vi "SP_Breakdown Summery Monthwise_.vi"() -> ()   [LabVIEW 2017]
uses:
  <vilib>/Math Plots/3D Math Plots/3D Pie/3D Pie XCtrl/3D Pie.xctl
  <vilib>/addons/database/Connection.llb/DB Tools Open Connec (Path).vi
  <vilib>/Math Plots/3D Math Plots/3D Pie/3D Pie Datatype/Public/Plot Helper (Vector).vi
  <vilib>/addons/database/NI_Database_API.lvlib
  <vilib>/Math Plots/3D Math Plots/3D Pie/3D Pie Datatype/3D Pie Datatype.lvclass
panel:
  in  "Cancel Button - Archive":bool
  in  "Get Rport 2":bool
  in  "Download 2":bool
  out "error out":errorcluster
  out "BD Count":string[][](array[string])
  out "Duration count":string[][](array[string])
  out "O/P 4":string[](array[string])
  out "month":string
  out "Table":string[][](array[string])
  out "Count":string[](array[string])
  out "Station ID":string[](array[string])
  out "Count out":string[](array[string])
  out "Elements Found out":string[](array[string])
  in  "Select Station":string(combo)
  in  "Shift":string(combo)
  out "T":string
  out "P":string
  out "Q":string
  out "M":string
  out "L":string
  out "GL":string
  in  "Select Year":string(combo)
  in  "Select Month":string(combo)
  in  "Tab Control":T1(tab)
  out "Table Control":string[][](table)
  out "heading 6":string="Total"
  out "heading 5":string="Production"
  out "heading 4":string="Qaulity"
  out "heading 3":string="Maintenance"
  out "heading2":string="Logistics"
  out "heading 1":string="Gap Leader"
  out "Count 2":refnum<class "3D Plot Datatype.lvclass">[](xcontrol)
  out "Duration":refnum<class "3D Plot Datatype.lvclass">[](xcontrol)
  # "Breakdown Summary Report (Month Wise)"
  # "L"
  # "M"
  # "S"
  # "M"
  # "Q"
  # "SS"
  # "TT"
  # "Designed And Developed By - Infinity Automation Systems Pvt. Ltd."
  # "Material"
  # "Safety"
  # "Maintenance"
  # "Quality"
  # "Total"
  # "Date"
  # "Startup/Setup"
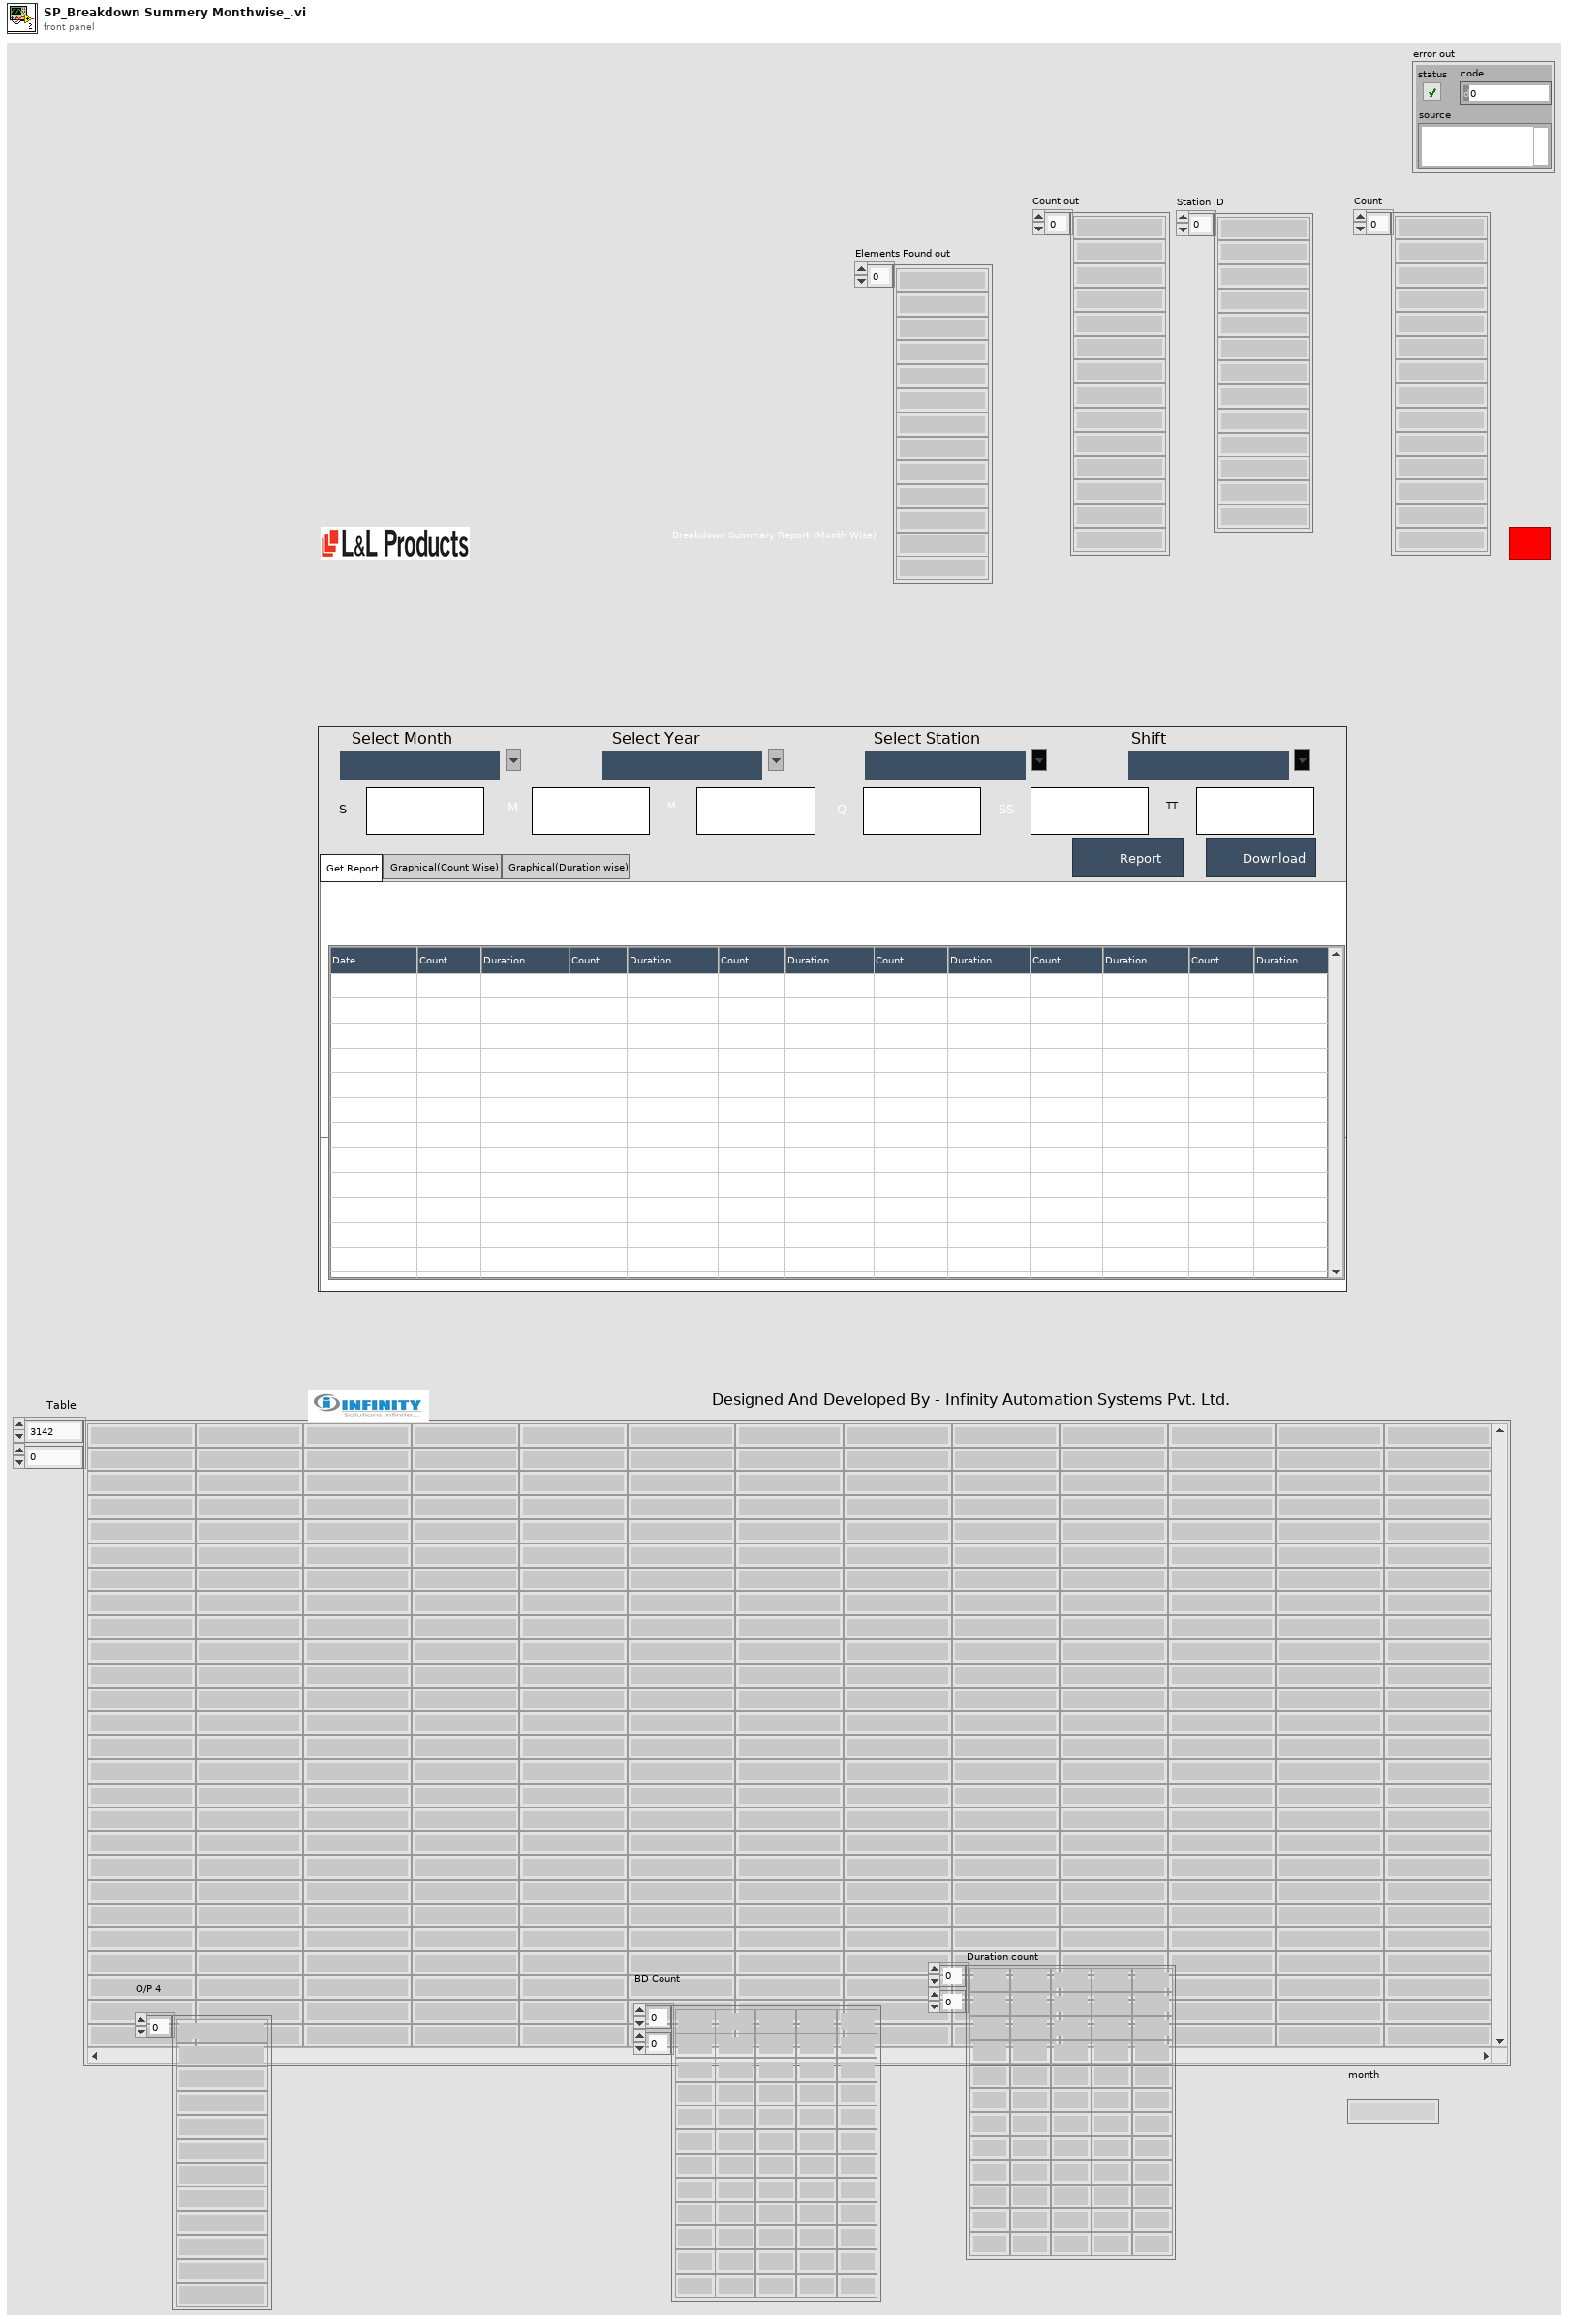
[diagram p1: front panel]
types:
  T1 = enum32{"Get Report", "Graphical(Count Wise) ", "Graphical(Duration wise)"}
  T2 = typedef "NI_Database_API.lvlib/Conn ObjectReference.ctl" = refnum<k1>
  T3 = enum32{"invalid app kind", "Development System", "Run Time System", "Student Edition", "Embedded LabVIEW", "Evaluation", "Custom"}
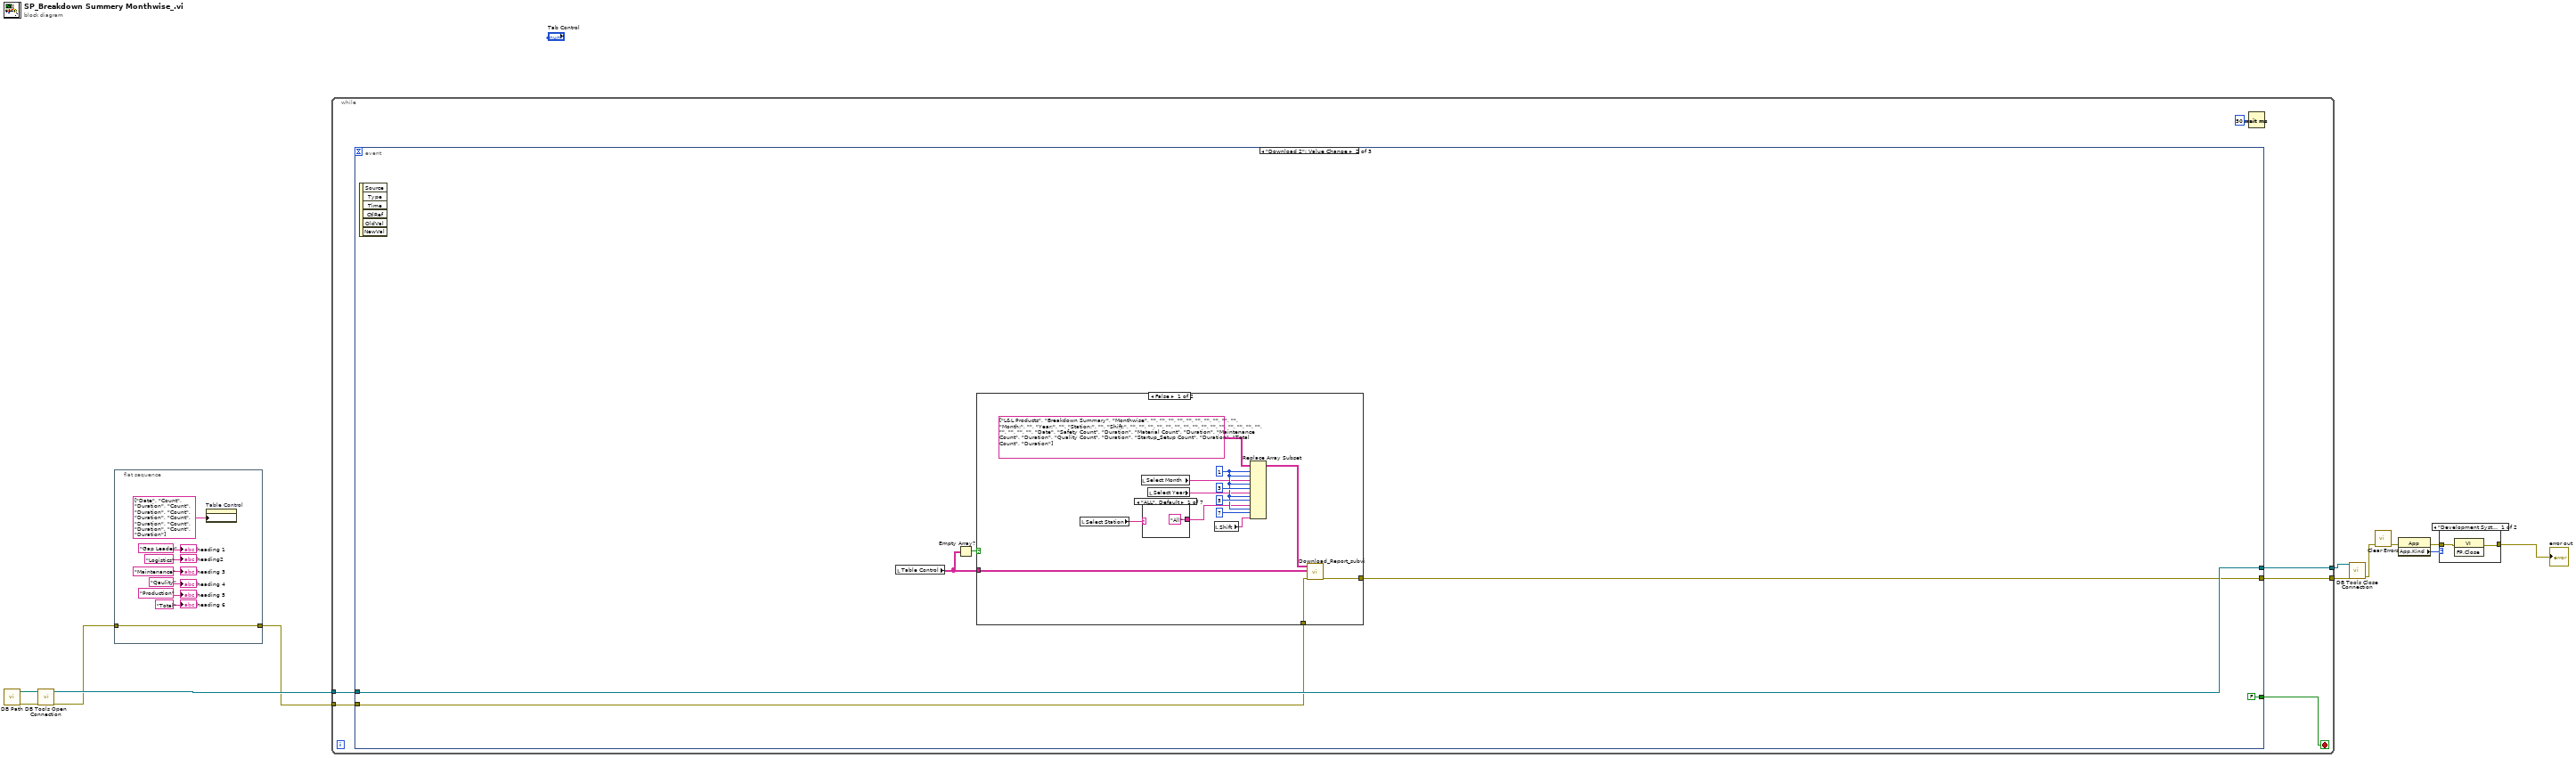
[diagram p0: block diagram]
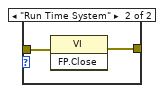
[diagram p2: hidden frame]
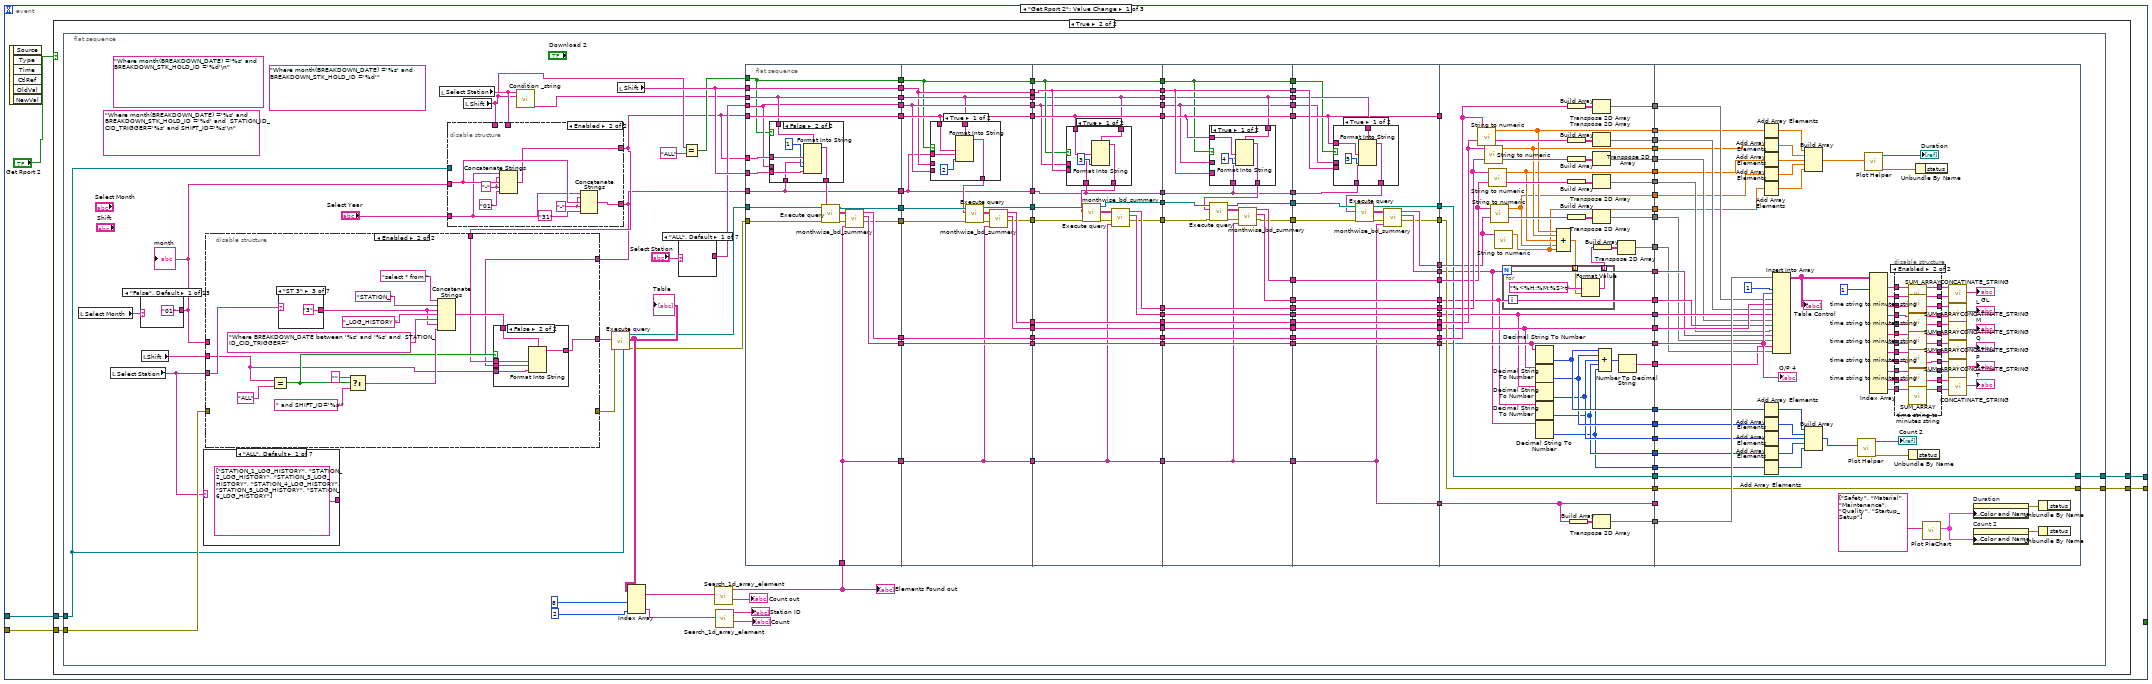
[diagram p3: hidden frame]
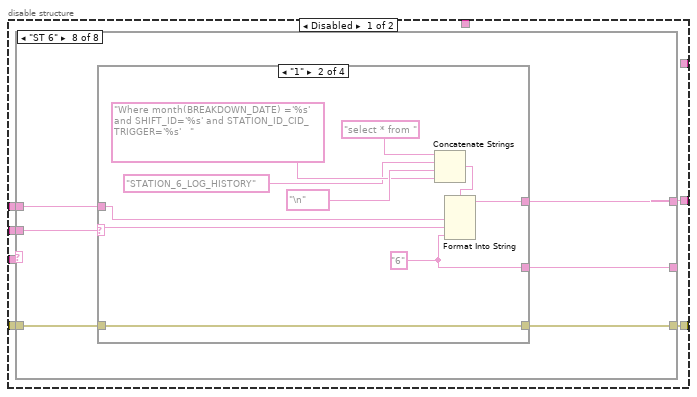
[diagram p5: hidden frame]
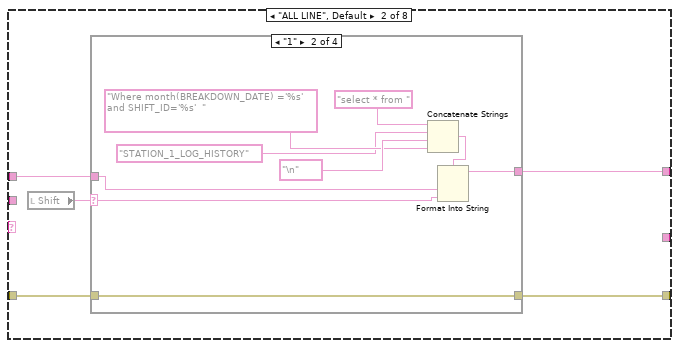
[diagram p7: hidden frame]
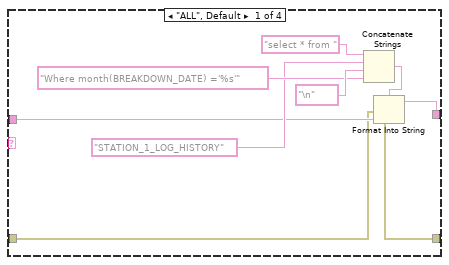
[diagram p8: hidden frame]
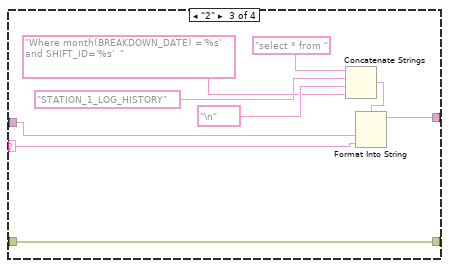
[diagram p9: hidden frame]
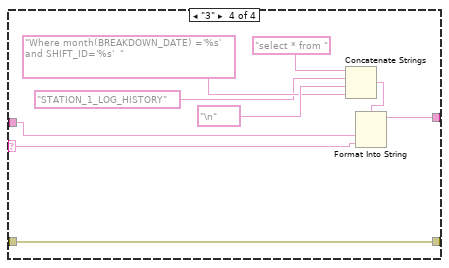
[diagram p10: hidden frame]
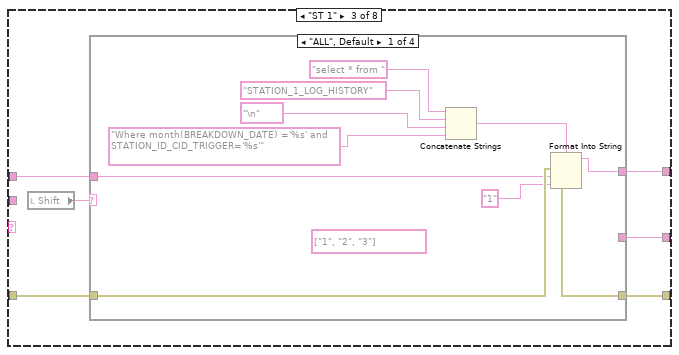
[diagram p11: hidden frame]
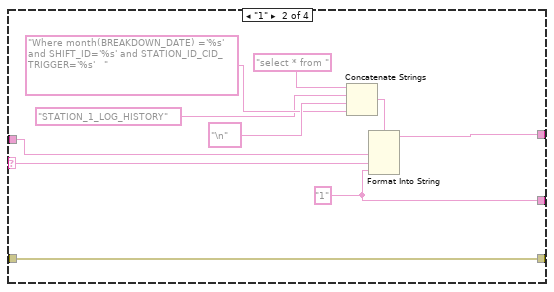
[diagram p12: hidden frame]
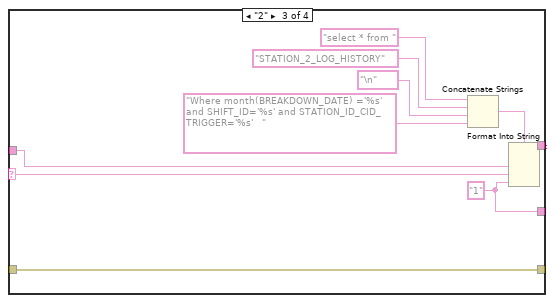
[diagram p13: hidden frame]
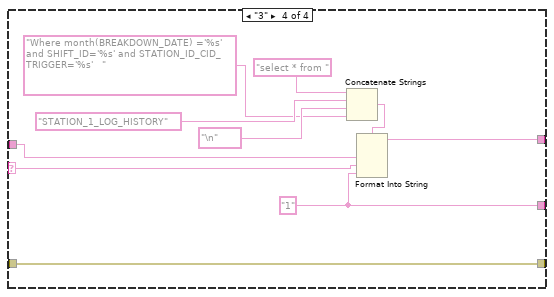
[diagram p14: hidden frame]
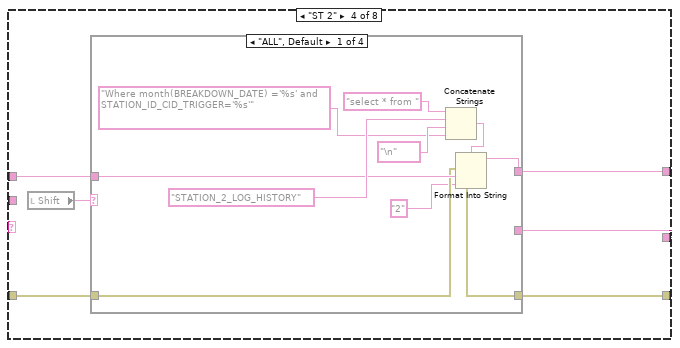
[diagram p15: hidden frame]
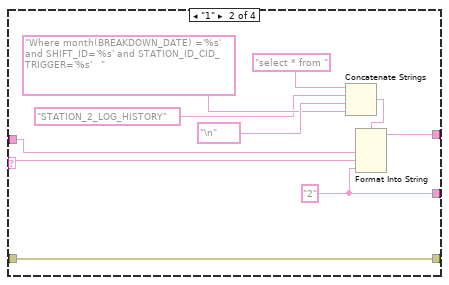
[diagram p16: hidden frame]
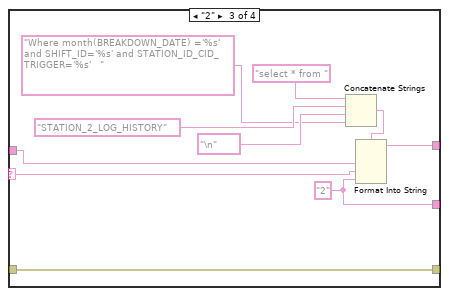
[diagram p17: hidden frame]
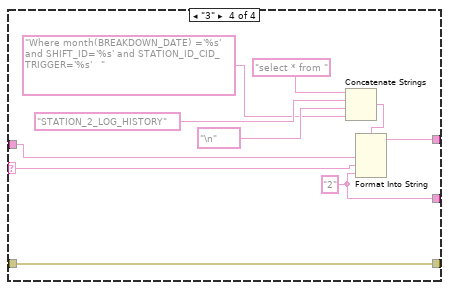
[diagram p18: hidden frame]
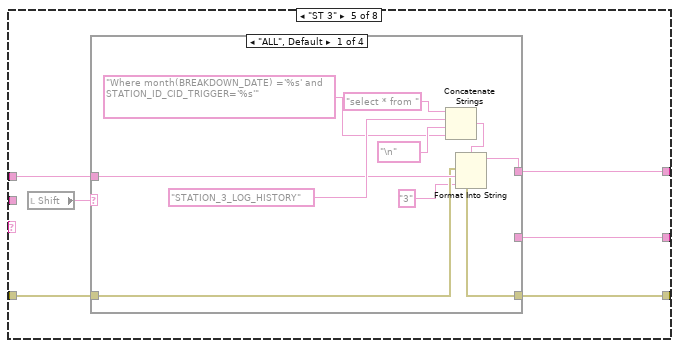
[diagram p19: hidden frame]
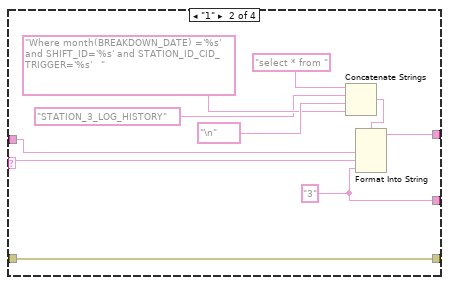
[diagram p20: hidden frame]
diagram:
  n1 = call "DB Path.vi"() -> ("error out"=w12:errorcluster, "DB Path"=w11:path)  [unwired: 10 in]
  n2 = call-poly <vilib>:"DB Tools Open Connection.vi"("error in (no error)"=w12, "connection information"=w11) -> ("error out"=w2:errorcluster, "connection reference"=w10:T2)  [unwired: 6 in]
  n3 = flat-sequence {
    tunnel: [w13] -> w1
    tunnel: w2 -> [w13]
    frame #0 {
      n4 = property on="Table Control" class="Tbl (strict)"("Column Headers[]"=string[] ["Date", "Count", "Duration", "Count", "Duration", "Count", "Duration", "Count", "Duration", "Count", "Duration", "Count", "Duration"] ("Column Header Strings[]")) -> ()  [unwired: 2 in, 2 out]
      "heading 1" <- "Gap Leader" ("heading 1")
      "heading2" <- "Logistics" ("heading2")
      "heading 3" <- "Maintenance" ("heading 3")
      "heading 4" <- "Qaulity" ("heading 4")
      "heading 5" <- "Production" ("heading 5")
      "heading 6" <- "Total" ("heading 6")
    }
  }
  n5 = while {
    tunnel: w1 -> [w26]
    tunnel: w10 -> [w25]
    tunnel: [w23] -> w4
    tunnel: [w22] -> w5
    stop <- w24 stop-if-true
    n6 = event shown="[1] \"Download 2\": Value Change" {
      selector: _ -> [_ _ _]
      dyn-events: _ -> [_ _ _]
      timeout: _ -> [_ _ _]
      tunnel: w26 -> [w31 w890 w917]
      tunnel: w25 -> [w30 w892 w916]
      tunnel: [_ FALSE ("Cancel Button - Archive") "Cancel Button - Archive"] -> w24
      tunnel: [w29 w889 w917] -> w23
      tunnel: [w28 w892 w916] -> w22
      event "Get Rport 2": Value Change {
        n7 = event-data() -> ()  [unwired: 1 in, 6 out]
        n8 = case shown="True" "Get Rport 2" {
          tunnel: w31 -> [_ w35]
          tunnel: w30 -> [_ w34]
          tunnel: [_ w33] -> w29
          tunnel: [_ w32] -> w28
          frame False {
          }
          frame True {
            n9 = flat-sequence {
              tunnel: w35 -> [w159]
              tunnel: w34 -> [w66]
              tunnel: [w63] -> w33
              tunnel: [w61] -> w32
              frame #0 {
                (unwired) "Where month(BREAKDOWN_DATE) ='%s' and  BREAKDOWN_STK_HOLD_ID ='%d' and  STATION_ID_CID_TRIGGER='%s' and SHIFT_ID='%s'\n" ("condition")
                (unwired) "Where month(BREAKDOWN_DATE) ='%s' and  BREAKDOWN_STK_HOLD_ID ='%d'" ("condition")
                (unwired) "Where month(BREAKDOWN_DATE) ='%s' and  BREAKDOWN_STK_HOLD_ID ='%d'\n" ("condition")
                n10 = local read "Select Month"() -> (w156:string)
                n11 = local read "Select Station"() -> (w57:string)
                n12 = case shown="\"False\", Default" w156 {
                  tunnel: ["01" "01" "02" "03" "04" "05" "06" "07" "08" "09" "10" "11" "12"] -> w65
                  frame "False", Default {
                  }
                  frame "January" {
                  }
                  frame "February" {
                  }
                  frame "March" {
                  }
                  frame "April" {
                  }
                  frame "May" {
                  }
                  frame "June" {
                  }
                  frame "July" {
                  }
                  frame "August" {
                  }
                  frame "September" {
                  }
                  frame "October" {
                  }
                  frame "November" {
                  }
                  frame "December" {
                  }
                }
                "month" <- w65
                n13 = local read "Shift"() -> (w48:string)
                n14 = case shown="\"ALL\", Default" w57 {
                  tunnel: [string[] ["STATION_1_LOG_HISTORY", "STATION_2_LOG_HISTORY", "STATION_3_LOG_HISTORY", "STATION_4_LOG_HISTORY", "STATION_5_LOG_HISTORY", "STATION_6_LOG_HISTORY"] string[] ["STATION_1_LOG_HISTORY"] string[] ["STATION_2_LOG_HISTORY"] string[] ["STATION_3_LOG_HISTORY"] string[] ["STATION_4_LOG_HISTORY"] string[] ["STATION_5_LOG_HISTORY"] string[] ["STATION_6_LOG_HISTORY"]] -> _
                  frame "ALL", Default {
                  }
                  frame "STATION 1" {
                  }
                  frame "STATION 2" {
                  }
                  frame "STATION 3" {
                  }
                  frame "STATION 4" {
                  }
                  frame "STATION 5" {
                  }
                  frame "STATION 6" {
                  }
                }
                n15 = local read "Select Station"() -> (w67:string)
                n16 = local read "Shift"() -> (w56:string)
                n17 = disable-structure shown="Enabled" {
                  disable-tunnel: w67 -> [w538 _]
                  disable-tunnel: w66 -> [w537 _]
                  disable-tunnel: w56 -> [w536 _]
                  disable-tunnel: w65 -> [w535 w546]
                  disable-tunnel: "Select Year" -> [w534 w539]
                  disable-tunnel: [_ w545] -> w47
                  disable-tunnel: [_ w544] -> w46
                  frame Disabled {
                    # "T=2\nF=4"
                    n18 = call "Condition _string_For_Month.vi"("Select Line 2"=w538, "connection reference"=w537, "Shift"=w536, "year"=w534, "month"=w535) -> ("Duration count"=→"Duration count":string[][], "BD Count"=→"BD Count":string[][])  [unwired: 11 in, 2 out]
                  }
                  frame Enabled {
                    w540 = "-" ("string")
                    w541 = "-" ("string")
                    n19 = Concatenate Strings(w539, w541, w546, w541, "01" ("string")) -> (w545:string)
                    n20 = Concatenate Strings(w539, w540, w546, w540, "31" ("string")) -> (w544:string)
                  }
                }
                n21 = disable-structure shown="Enabled" {
                  disable-tunnel: [w169 w487] -> w163
                  disable-tunnel: w159 -> [w168 _]
                  disable-tunnel: [w167 _] -> w158
                  disable-tunnel: w65 -> [w166 _]
                  disable-tunnel: w57 -> [w165 w494]
                  disable-tunnel: w48 -> [w164 w488]
                  disable-tunnel: w47 -> [_ w490]
                  disable-tunnel: w46 -> [_ w489]
                  frame Disabled {
                    n22 = case shown="\"ST 6\"" w165 {
                      tunnel: w166 -> [_ w174 w216 w262 w308 w354 w400 w446]
                      tunnel: [_ w173 w215 w261 w307 w353 w399 w445] -> w169
                      tunnel: w168 -> [_ w172 w214 w260 w306 w352 w398 w444]
                      tunnel: [_ w171 w213 w259 w305 w351 w397 w443] -> w167
                      tunnel: [_ _ w211 w257 w303 w349 w395 w442] -> _
                      tunnel: w164 -> [_ _ _ _ _ _ _ w441]
                      frame "False" {
                      }
                      frame "ALL LINE", Default {
                        n23 = local read "Shift"() -> (w170:string)
                        n24 = case shown="\"1\"" w170 {
                          selector: w170 -> [_ w185 w194 w203]
                          tunnel: [w179 w188 w197 w206] -> w173
                          tunnel: [w178 w184 w193 w202] -> w171
                          tunnel: w174 -> [w176 w186 w195 w204]
                          tunnel: w172 -> [w175 w184 w193 w202]
                          frame "ALL", Default {
                            n25 = Concatenate Strings("select * from " ("string"), "STATION_1_LOG_HISTORY" ("table"), "\n" ("string"), "Where month(BREAKDOWN_DATE) ='%s'" ("condition")) -> (w180:string)
                            n26 = Format Into String(format string=w180, error in=w175, w176) -> (resulting string=w179:string, error out=w178:errorcluster)  [unwired: 1 in]
                          }
                          frame "1" {
                            n27 = Concatenate Strings("select * from " ("string"), "STATION_1_LOG_HISTORY" ("table"), "\n" ("string"), "Where month(BREAKDOWN_DATE) ='%s' and SHIFT_ID='%s'  " ("condition")) -> (w190:string)
                            n28 = Format Into String(format string=w190, w186, w185) -> (resulting string=w188:string)  [unwired: 2 in, 1 out]
                          }
                          frame "2" {
                            n29 = Concatenate Strings("select * from " ("string"), "STATION_1_LOG_HISTORY" ("table"), "\n" ("string"), "Where month(BREAKDOWN_DATE) ='%s' and SHIFT_ID='%s'  " ("condition")) -> (w199:string)
                            n30 = Format Into String(format string=w199, w195, w194) -> (resulting string=w197:string)  [unwired: 2 in, 1 out]
                          }
                          frame "3" {
                            n31 = Concatenate Strings("select * from " ("string"), "STATION_1_LOG_HISTORY" ("table"), "\n" ("string"), "Where month(BREAKDOWN_DATE) ='%s' and SHIFT_ID='%s'  " ("condition")) -> (w208:string)
                            n32 = Format Into String(format string=w208, w204, w203) -> (resulting string=w206:string)  [unwired: 2 in, 1 out]
                          }
                        }
                      }
                      frame "ST 1" {
                        n33 = local read "Shift"() -> (w212:string)
                        n34 = case shown="\"ALL\", Default" w212 {
                          selector: w212 -> [_ w230 w240 w250]
                          tunnel: [w222 w233 w243 w253] -> w215
                          tunnel: [w221 w229 w239 w249] -> w213
                          tunnel: w216 -> [w217 w231 w241 w251]
                          tunnel: w214 -> [w219 w229 w239 w249]
                          tunnel: [_ w227 w237 w247] -> w211
                          frame "ALL", Default {
                            (unwired) string[] ["1", "2", "3"]
                            n35 = Concatenate Strings("select * from " ("string"), "STATION_1_LOG_HISTORY" ("table"), "\n" ("string"), "Where month(BREAKDOWN_DATE) ='%s' and  STATION_ID_CID_TRIGGER='%s'" ("condition")) -> (w223:string)
                            n36 = Format Into String(format string=w223, error in=w219, w217, "1") -> (resulting string=w222:string, error out=w221:errorcluster)  [unwired: 1 in]
                          }
                          frame "1" {
                            w227 = "1"
                            n37 = Concatenate Strings("select * from " ("string"), "STATION_1_LOG_HISTORY" ("table"), "\n" ("string"), "Where month(BREAKDOWN_DATE) ='%s' and SHIFT_ID='%s' and STATION_ID_CID_TRIGGER='%s'   " ("condition")) -> (w228:string)
                            n38 = Format Into String(format string=w228, w231, w230, w227) -> (resulting string=w233:string)  [unwired: 2 in, 1 out]
                          }
                          frame "2" {
                            w237 = "1" ("input 3")
                            n39 = Concatenate Strings("select * from " ("string"), "STATION_2_LOG_HISTORY" ("table"), "\n" ("string"), "Where month(BREAKDOWN_DATE) ='%s' and SHIFT_ID='%s' and STATION_ID_CID_TRIGGER='%s'   " ("condition")) -> (w244:string)
                            n40 = Format Into String(format string=w244, w241, w240, w237) -> (resulting string=w243:string)  [unwired: 2 in, 1 out]
                          }
                          frame "3" {
                            w247 = "1" ("input 3")
                            n41 = Concatenate Strings("select * from " ("string"), "STATION_1_LOG_HISTORY" ("table"), "\n" ("string"), "Where month(BREAKDOWN_DATE) ='%s' and SHIFT_ID='%s' and STATION_ID_CID_TRIGGER='%s'   " ("condition")) -> (w254:string)
                            n42 = Format Into String(format string=w254, w251, w250, w247) -> (resulting string=w253:string)  [unwired: 2 in, 1 out]
                          }
                        }
                      }
                      frame "ST 2" {
                        n43 = local read "Shift"() -> (w258:string)
                        n44 = case shown="\"ALL\", Default" w258 {
                          selector: w258 -> [_ w275 w286 w296]
                          tunnel: [w269 w278 w289 w299] -> w261
                          tunnel: [w268 w274 w285 w295] -> w259
                          tunnel: w262 -> [w266 w276 w287 w297]
                          tunnel: w260 -> [w265 w274 w285 w295]
                          tunnel: [_ w273 w283 w293] -> w257
                          frame "ALL", Default {
                            n45 = Concatenate Strings("select * from " ("string"), "STATION_2_LOG_HISTORY" ("table"), "\n" ("string"), "Where month(BREAKDOWN_DATE) ='%s' and  STATION_ID_CID_TRIGGER='%s'" ("condition")) -> (w270:string)
                            n46 = Format Into String(format string=w270, error in=w265, w266, "2" ("input 2")) -> (resulting string=w269:string, error out=w268:errorcluster)  [unwired: 1 in]
                          }
                          frame "1" {
                            w273 = "2"
                            n47 = Concatenate Strings("select * from " ("string"), "STATION_2_LOG_HISTORY" ("table"), "\n" ("string"), "Where month(BREAKDOWN_DATE) ='%s' and SHIFT_ID='%s' and STATION_ID_CID_TRIGGER='%s'   " ("condition")) -> (w280:string)
                            n48 = Format Into String(format string=w280, w276, w275, w273) -> (resulting string=w278:string)  [unwired: 2 in, 1 out]
                          }
                          frame "2" {
                            w283 = "2" ("input 3")
                            n49 = Concatenate Strings("select * from " ("string"), "STATION_2_LOG_HISTORY" ("table"), "\n" ("string"), "Where month(BREAKDOWN_DATE) ='%s' and SHIFT_ID='%s' and STATION_ID_CID_TRIGGER='%s'   " ("condition")) -> (w290:string)
                            n50 = Format Into String(format string=w290, w287, w286, w283) -> (resulting string=w289:string)  [unwired: 2 in, 1 out]
                          }
                          frame "3" {
                            w293 = "2" ("input 3")
                            n51 = Concatenate Strings("select * from " ("string"), "STATION_2_LOG_HISTORY" ("table"), "\n" ("string"), "Where month(BREAKDOWN_DATE) ='%s' and SHIFT_ID='%s' and STATION_ID_CID_TRIGGER='%s'   " ("condition")) -> (w300:string)
                            n52 = Format Into String(format string=w300, w297, w296, w293) -> (resulting string=w299:string)  [unwired: 2 in, 1 out]
                          }
                        }
                      }
                      frame "ST 3" {
                        n53 = local read "Shift"() -> (w304:string)
                        n54 = case shown="\"ALL\", Default" w304 {
                          selector: w304 -> [_ w321 w332 w342]
                          tunnel: [w315 w324 w335 w345] -> w307
                          tunnel: [w314 w320 w331 w341] -> w305
                          tunnel: w308 -> [w312 w322 w333 w343]
                          tunnel: w306 -> [w311 w320 w331 w341]
                          tunnel: [_ w319 w329 w339] -> w303
                          frame "ALL", Default {
                            n55 = Concatenate Strings("select * from " ("string"), "STATION_3_LOG_HISTORY" ("table"), "\n" ("string"), "Where month(BREAKDOWN_DATE) ='%s' and  STATION_ID_CID_TRIGGER='%s'" ("condition")) -> (w316:string)
                            n56 = Format Into String(format string=w316, error in=w311, w312, "3" ("input 2")) -> (resulting string=w315:string, error out=w314:errorcluster)  [unwired: 1 in]
                          }
                          frame "1" {
                            w319 = "3"
                            n57 = Concatenate Strings("select * from " ("string"), "STATION_3_LOG_HISTORY" ("table"), "\n" ("string"), "Where month(BREAKDOWN_DATE) ='%s' and SHIFT_ID='%s' and STATION_ID_CID_TRIGGER='%s'   " ("condition")) -> (w326:string)
                            n58 = Format Into String(format string=w326, w322, w321, w319) -> (resulting string=w324:string)  [unwired: 2 in, 1 out]
                          }
                          frame "2" {
                            w329 = "3" ("input 3")
                            n59 = Concatenate Strings("select * from " ("string"), "STATION_3_LOG_HISTORY" ("table"), "\n" ("string"), "Where month(BREAKDOWN_DATE) ='%s' and SHIFT_ID='%s' and STATION_ID_CID_TRIGGER='%s'   " ("condition")) -> (w336:string)
                            n60 = Format Into String(format string=w336, w333, w332, w329) -> (resulting string=w335:string)  [unwired: 2 in, 1 out]
                          }
                          frame "3" {
                            w339 = "3" ("input 3")
                            n61 = Concatenate Strings("select * from " ("string"), "STATION_3_LOG_HISTORY" ("table"), "\n" ("string"), "Where month(BREAKDOWN_DATE) ='%s' and SHIFT_ID='%s' and STATION_ID_CID_TRIGGER='%s'   " ("condition")) -> (w346:string)
                            n62 = Format Into String(format string=w346, w343, w342, w339) -> (resulting string=w345:string)  [unwired: 2 in, 1 out]
                          }
                        }
                      }
                      frame "ST 4" {
                        n63 = local read "Shift"() -> (w350:string)
                        n64 = case shown="\"ALL\", Default" w350 {
                          selector: w350 -> [_ w367 w378 w388]
                          tunnel: [w361 w370 w381 w391] -> w353
                          tunnel: [w360 w366 w377 w387] -> w351
                          tunnel: w354 -> [w358 w368 w379 w389]
                          tunnel: w352 -> [w357 w366 w377 w387]
                          tunnel: [_ w365 w375 w385] -> w349
                          frame "ALL", Default {
                            n65 = Concatenate Strings("select * from " ("string"), "STATION_4_LOG_HISTORY" ("table"), "\n" ("string"), "Where month(BREAKDOWN_DATE) ='%s' and  STATION_ID_CID_TRIGGER='%s'" ("condition")) -> (w362:string)
                            n66 = Format Into String(format string=w362, error in=w357, w358, "4" ("input 2")) -> (resulting string=w361:string, error out=w360:errorcluster)  [unwired: 1 in]
                          }
                          frame "1" {
                            w365 = "4"
                            n67 = Concatenate Strings("select * from " ("string"), "STATION_4_LOG_HISTORY" ("table"), "\n" ("string"), "Where month(BREAKDOWN_DATE) ='%s' and SHIFT_ID='%s' and STATION_ID_CID_TRIGGER='%s'   " ("condition")) -> (w372:string)
                            n68 = Format Into String(format string=w372, w368, w367, w365) -> (resulting string=w370:string)  [unwired: 2 in, 1 out]
                          }
                          frame "2" {
                            w375 = "4" ("input 3")
                            n69 = Concatenate Strings("select * from " ("string"), "STATION_4_LOG_HISTORY" ("table"), "\n" ("string"), "Where month(BREAKDOWN_DATE) ='%s' and SHIFT_ID='%s' and STATION_ID_CID_TRIGGER='%s'   " ("condition")) -> (w382:string)
                            n70 = Format Into String(format string=w382, w379, w378, w375) -> (resulting string=w381:string)  [unwired: 2 in, 1 out]
                          }
                          frame "3" {
                            w385 = "4" ("input 3")
                            n71 = Concatenate Strings("select * from " ("string"), "STATION_4_LOG_HISTORY" ("table"), "\n" ("string"), "Where month(BREAKDOWN_DATE) ='%s' and SHIFT_ID='%s' and STATION_ID_CID_TRIGGER='%s'   " ("condition")) -> (w392:string)
                            n72 = Format Into String(format string=w392, w389, w388, w385) -> (resulting string=w391:string)  [unwired: 2 in, 1 out]
                          }
                        }
                      }
                      frame "ST 5" {
                        n73 = local read "Shift"() -> (w396:string)
                        n74 = case shown="\"ALL\", Default" w396 {
                          selector: w396 -> [_ w413 w424 w434]
                          tunnel: [w407 w416 w427 w437] -> w399
                          tunnel: [w406 w412 w423 w433] -> w397
                          tunnel: w400 -> [w404 w414 w425 w435]
                          tunnel: w398 -> [w403 w412 w423 w433]
                          tunnel: [_ w411 w421 w431] -> w395
                          frame "ALL", Default {
                            n75 = Concatenate Strings("select * from " ("string"), "STATION_5_LOG_HISTORY" ("table"), "\n" ("string"), "Where month(BREAKDOWN_DATE) ='%s' and  STATION_ID_CID_TRIGGER='%s'" ("condition")) -> (w408:string)
                            n76 = Format Into String(format string=w408, error in=w403, w404, "5" ("input 2")) -> (resulting string=w407:string, error out=w406:errorcluster)  [unwired: 1 in]
                          }
                          frame "1" {
                            w411 = "5"
                            n77 = Concatenate Strings("select * from " ("string"), "STATION_5_LOG_HISTORY" ("table"), "\n" ("string"), "Where month(BREAKDOWN_DATE) ='%s' and SHIFT_ID='%s' and STATION_ID_CID_TRIGGER='%s'   " ("condition")) -> (w418:string)
                            n78 = Format Into String(format string=w418, w414, w413, w411) -> (resulting string=w416:string)  [unwired: 2 in, 1 out]
                          }
                          frame "2" {
                            w421 = "5" ("input 3")
                            n79 = Concatenate Strings("select * from " ("string"), "STATION_5_LOG_HISTORY" ("table"), "\n" ("string"), "Where month(BREAKDOWN_DATE) ='%s' and SHIFT_ID='%s' and STATION_ID_CID_TRIGGER='%s'   " ("condition")) -> (w428:string)
                            n80 = Format Into String(format string=w428, w425, w424, w421) -> (resulting string=w427:string)  [unwired: 2 in, 1 out]
                          }
                          frame "3" {
                            w431 = "5" ("input 3")
                            n81 = Concatenate Strings("select * from " ("string"), "STATION_5_LOG_HISTORY" ("table"), "\n" ("string"), "Where month(BREAKDOWN_DATE) ='%s' and SHIFT_ID='%s' and STATION_ID_CID_TRIGGER='%s'   " ("condition")) -> (w438:string)
                            n82 = Format Into String(format string=w438, w435, w434, w431) -> (resulting string=w437:string)  [unwired: 2 in, 1 out]
                          }
                        }
                      }
                      frame "ST 6" {
                        n83 = case shown="\"1\"" w441 {
                          selector: w441 -> [_ w459 w470 w480]
                          tunnel: [w453 w462 w473 w483] -> w445
                          tunnel: [w452 w458 w469 w479] -> w443
                          tunnel: w446 -> [w450 w460 w471 w481]
                          tunnel: w444 -> [w449 w458 w469 w479]
                          tunnel: [_ w457 w467 w477] -> w442
                          frame "ALL", Default {
                            n84 = Concatenate Strings("select * from " ("string"), "STATION_6_LOG_HISTORY" ("table"), "\n" ("string"), "Where month(BREAKDOWN_DATE) ='%s' and  STATION_ID_CID_TRIGGER='%s'" ("condition")) -> (w454:string)
                            n85 = Format Into String(format string=w454, error in=w449, w450, "6" ("input 2")) -> (resulting string=w453:string, error out=w452:errorcluster)  [unwired: 1 in]
                          }
                          frame "1" {
                            w457 = "6"
                            n86 = Concatenate Strings("select * from " ("string"), "STATION_6_LOG_HISTORY" ("table"), "\n" ("string"), "Where month(BREAKDOWN_DATE) ='%s' and SHIFT_ID='%s' and STATION_ID_CID_TRIGGER='%s'   " ("condition")) -> (w464:string)
                            n87 = Format Into String(format string=w464, w460, w459, w457) -> (resulting string=w462:string)  [unwired: 2 in, 1 out]
                          }
                          frame "2" {
                            w467 = "6" ("input 3")
                            n88 = Concatenate Strings("select * from " ("string"), "STATION_6_LOG_HISTORY" ("table"), "\n" ("string"), "Where month(BREAKDOWN_DATE) ='%s' and SHIFT_ID='%s' and STATION_ID_CID_TRIGGER='%s'   " ("condition")) -> (w474:string)
                            n89 = Format Into String(format string=w474, w471, w470, w467) -> (resulting string=w473:string)  [unwired: 2 in, 1 out]
                          }
                          frame "3" {
                            w477 = "6" ("input 3")
                            n90 = Concatenate Strings("select * from " ("string"), "STATION_6_LOG_HISTORY" ("table"), "\n" ("string"), "Where month(BREAKDOWN_DATE) ='%s' and SHIFT_ID='%s' and STATION_ID_CID_TRIGGER='%s'   " ("condition")) -> (w484:string)
                            n91 = Format Into String(format string=w484, w481, w480, w477) -> (resulting string=w483:string)  [unwired: 2 in, 1 out]
                          }
                        }
                      }
                    }
                  }
                  frame Enabled {
                    n92 = Equal?(x=w488, y="ALL" ("condition")) -> (x = y?=w492:bool)
                    n93 = case shown="\"ST 3\"" w494 {
                      tunnel: ["1" "2" "3" "4" "5" "6" "1"] -> w493
                      frame "ST 1" {
                      }
                      frame "ST 2" {
                      }
                      frame "ST 3" {
                      }
                      frame "ST 4" {
                      }
                      frame "ST 5" {
                      }
                      frame "ST 6" {
                      }
                      frame "ALL", Default {
                      }
                    }
                    n94 = Select(t="", s=w492, f=" and SHIFT_ID='%s'" ("condition")) -> (s? t:f=w502:string)
                    n95 = Concatenate Strings("select * from " ("string"), "STATION_" ("table"), w493, "_LOG_HISTORY " ("table"), "Where BREAKDOWN_DATE between '%s' and '%s' and  STATION_ID_CID_TRIGGER=" ("condition"), w493, w502) -> (w491:string)
                    n96 = case shown="False" w492 {
                      tunnel: w490 -> [w506 w511]
                      tunnel: w491 -> [w505 w510]
                      tunnel: [w504 w509] -> w487
                      tunnel: w489 -> [w503 w508]
                      tunnel: w488 -> [_ w507]
                      frame True {
                        n97 = Format Into String(format string=w505, w506, w503) -> (resulting string=w504:string)  [unwired: 2 in, 1 out]
                      }
                      frame False {
                        n98 = Format Into String(format string=w510, w511, w508, w507) -> (resulting string=w509:string)  [unwired: 2 in, 1 out]
                      }
                    }
                  }
                }
                n99 = call "Condition _string.vi"("Shift"=w56, "Select Line 2"=w67) -> ("String"=w53:string)  [unwired: 7 in, 2 out]
                n100 = call "Execute query.vi"("error in (no error)"=w158, "String"=w163, "connection reference"=w66) -> ("error out"=w151:errorcluster, "Table"=w161:string[][], "connection reference 2"=w150:T2)  [unwired: 5 in, 1 out]
                "Table" <- w161
                n101 = local read "Shift"() -> (w78:string)
                n102 = Index Array(array=w161, index (col) #1=8 ("disabled index (col)"), index (col) #2=2 ("index (col)")) -> (element #1=w162:string[], element #2=w154:string[])  [unwired: 2 in]
                n103 = case shown="\"ALL\", Default" "Select Station" {
                  tunnel: [_ "1" "2" "3" "4" "5" "6"] -> w58
                  frame "ALL", Default {
                  }
                  frame "ST 1" {
                  }
                  frame "ST 2" {
                  }
                  frame "ST 3" {
                  }
                  frame "ST 4" {
                  }
                  frame "ST 5" {
                  }
                  frame "ST 6" {
                  }
                }
                n104 = Equal?(x=w56, y="ALL") -> (x = y?=w54:bool)
                n105 = call "Search_1d_array_element.vi"("BD Date"=w162) -> ("Count out"=→"Count out":string[], "Elements Found out"=w91:string[])  [unwired: 6 in, 1 out]
                "Elements Found out" <- w91
                n106 = call "Search_1d_array_element.vi"("BD Date"=w154) -> ("Count out"=→"Count":string[], "Elements Found out"=→"Station ID":string[])  [unwired: 6 in, 1 out]
                n107 = flat-sequence {
                  tunnel: w151 -> [w564]
                  tunnel: w150 -> [w563]
                  tunnel: w47 -> [w561]
                  tunnel: [w560] -> w149
                  tunnel: w47 -> [w560]
                  tunnel: [w559] -> w148
                  tunnel: [w558] -> w147
                  tunnel: [w557] -> w146
                  tunnel: [w555] -> w145
                  tunnel: w91 -> [w554]
                  tunnel: [w554] -> w90
                  tunnel: w58 -> [w552]
                  tunnel: [w552] -> w85
                  tunnel: w53 -> [w553]
                  tunnel: [w553] -> w83
                  tunnel: w78 -> [w551]
                  tunnel: [w550] -> w79
                  tunnel: w78 -> [w550]
                  tunnel: w54 -> [w548]
                  tunnel: [w548] -> w73
                  tunnel: w46 -> [w547]
                  tunnel: [w547] -> w52
                  tunnel: w149 -> [w582]
                  tunnel: w148 -> [w592]
                  tunnel: w147 -> [w587]
                  tunnel: w146 -> [w588]
                  tunnel: w145 -> [w591]
                  tunnel: [w588] -> w144
                  tunnel: [w587] -> w143
                  tunnel: [w586] -> w142
                  tunnel: [w585] -> w141
                  tunnel: [w584] -> w140
                  tunnel: [w583] -> w139
                  tunnel: [w582] -> w122
                  tunnel: w90 -> [w581]
                  tunnel: [w581] -> w89
                  tunnel: w85 -> [w580]
                  tunnel: [w580] -> w84
                  tunnel: w83 -> [w579]
                  tunnel: [w579] -> w82
                  tunnel: w79 -> [w578]
                  tunnel: [w578] -> w77
                  tunnel: w73 -> [w577]
                  tunnel: [w577] -> w72
                  tunnel: w52 -> [w576]
                  tunnel: [w576] -> w51
                  tunnel: w144 -> [w624]
                  tunnel: w143 -> [w623]
                  tunnel: w142 -> [w622]
                  tunnel: w141 -> [w621]
                  tunnel: w140 -> [w618]
                  tunnel: w139 -> [w617]
                  tunnel: [w624] -> w138
                  tunnel: [w623] -> w137
                  tunnel: [w622] -> w136
                  tunnel: [w621] -> w135
                  tunnel: [w616] -> w134
                  tunnel: [w615] -> w133
                  tunnel: [w614] -> w132
                  tunnel: [w613] -> w131
                  tunnel: w122 -> [w611]
                  tunnel: [w611] -> w121
                  tunnel: w89 -> [w612]
                  tunnel: [w612] -> w88
                  tunnel: w84 -> [w607]
                  tunnel: w82 -> [w606]
                  tunnel: [w606] -> w81
                  tunnel: w77 -> [w610]
                  tunnel: [w610] -> w76
                  tunnel: w72 -> [w608]
                  tunnel: [w608] -> w71
                  tunnel: [w607] -> w70
                  tunnel: w51 -> [w605]
                  tunnel: [w605] -> w50
                  tunnel: w138 -> [w657]
                  tunnel: w137 -> [w656]
                  tunnel: w136 -> [w655]
                  tunnel: w135 -> [w654]
                  tunnel: w134 -> [w653]
                  tunnel: w133 -> [w652]
                  tunnel: w132 -> [w649]
                  tunnel: w131 -> [w648]
                  tunnel: [w657] -> w130
                  tunnel: [w656] -> w129
                  tunnel: [w655] -> w128
                  tunnel: [w654] -> w127
                  tunnel: [w653] -> w126
                  tunnel: [w652] -> w125
                  tunnel: [w647] -> w124
                  tunnel: [w646] -> w123
                  tunnel: w121 -> [w641]
                  tunnel: [w645] -> w120
                  tunnel: [w644] -> w119
                  tunnel: [w641] -> w118
                  tunnel: w88 -> [w643]
                  tunnel: [w643] -> w87
                  tunnel: w81 -> [w639]
                  tunnel: [w639] -> w80
                  tunnel: w76 -> [w642]
                  tunnel: [w642] -> w75
                  tunnel: w71 -> [w637]
                  tunnel: w70 -> [w638]
                  tunnel: [w638] -> w69
                  tunnel: [w637] -> w68
                  tunnel: w50 -> [w636]
                  tunnel: [w636] -> w49
                  tunnel: w130 -> [w692]
                  tunnel: w129 -> [w691]
                  tunnel: w128 -> [w690]
                  tunnel: w127 -> [w689]
                  tunnel: w126 -> [w688]
                  tunnel: w125 -> [w687]
                  tunnel: w124 -> [w686]
                  tunnel: w123 -> [w685]
                  tunnel: w120 -> [w682]
                  tunnel: w119 -> [w681]
                  tunnel: w118 -> [w672]
                  tunnel: [w692] -> w117
                  tunnel: [w691] -> w116
                  tunnel: [w690] -> w115
                  tunnel: [w689] -> w114
                  tunnel: [w688] -> w113
                  tunnel: [w687] -> w112
                  tunnel: [w686] -> w111
                  tunnel: [w685] -> w110
                  tunnel: [w680] -> w109
                  tunnel: [w679] -> w108
                  tunnel: [w678] -> w107
                  tunnel: [w677] -> w106
                  tunnel: [w672] -> w105
                  tunnel: w87 -> [w676]
                  tunnel: [w676] -> w86
                  tunnel: w80 -> [w673]
                  tunnel: w75 -> [w674]
                  tunnel: w69 -> [w671]
                  tunnel: w68 -> [w670]
                  tunnel: w49 -> [w669]
                  tunnel: w117 -> [w738]
                  tunnel: w116 -> [w713]
                  tunnel: w115 -> [w712]
                  tunnel: w114 -> [w737]
                  tunnel: w113 -> [w711]
                  tunnel: w112 -> [w736]
                  tunnel: w111 -> [w710]
                  tunnel: w110 -> [w735]
                  tunnel: w109 -> [w709]
                  tunnel: w108 -> [w734]
                  tunnel: w107 -> [w721]
                  tunnel: w106 -> [w722]
                  tunnel: w105 -> [_]
                  tunnel: [w731] -> w104
                  tunnel: [w713] -> w103
                  tunnel: [w730] -> w102
                  tunnel: [w712] -> w101
                  tunnel: [w729] -> w100
                  tunnel: [w711] -> w99
                  tunnel: [w728] -> w98
                  tunnel: [w710] -> w97
                  tunnel: [w727] -> w96
                  tunnel: [w709] -> w95
                  tunnel: [w726] -> w94
                  tunnel: [w725] -> w93
                  tunnel: [w724] -> w92
                  tunnel: w86 -> [w723]
                  tunnel: [w723] -> w74
                  tunnel: [w722] -> w62
                  tunnel: [w721] -> w60
                  tunnel: [w718] -> w45
                  tunnel: [w717] -> w44
                  tunnel: [w716] -> w43
                  tunnel: [w715] -> w42
                  tunnel: [w714] -> w41
                  tunnel: [w708] -> w40
                  tunnel: [w707] -> w39
                  tunnel: [w706] -> w38
                  tunnel: [w705] -> w37
                  tunnel: [w704] -> w36
                  tunnel: w104 -> [w824]
                  tunnel: w103 -> [w823]
                  tunnel: w102 -> [w822]
                  tunnel: w101 -> [w821]
                  tunnel: w100 -> [w820]
                  tunnel: w99 -> [w819]
                  tunnel: w98 -> [w818]
                  tunnel: w97 -> [w817]
                  tunnel: w96 -> [w816]
                  tunnel: w95 -> [w815]
                  tunnel: w94 -> [w814]
                  tunnel: w93 -> [w812]
                  tunnel: w92 -> [w813]
                  tunnel: w74 -> [_]
                  tunnel: [w779] -> w63
                  tunnel: w62 -> [w779]
                  tunnel: [w778] -> w61
                  tunnel: w60 -> [w778]
                  tunnel: w45 -> [w757]
                  tunnel: w44 -> [w756]
                  tunnel: w43 -> [w755]
                  tunnel: w42 -> [w754]
                  tunnel: w41 -> [w753]
                  tunnel: w40 -> [w752]
                  tunnel: w39 -> [w751]
                  tunnel: w38 -> [w750]
                  tunnel: w37 -> [w749]
                  tunnel: w36 -> [w748]
                  frame #0 {
                    n108 = case shown="False" w548 {
                      tunnel: w561 -> [w569 w575]
                      tunnel: w553 -> [w567 w573]
                      tunnel: w552 -> [_ _]
                      tunnel: w551 -> [_ w572]
                      tunnel: [w566 w571] -> w549
                      tunnel: w547 -> [w565 w570]
                      frame True {
                        n109 = Format Into String(format string=w567, w569, w565, 1 ("BREAKDOWN_STK_HOLD_ID")) -> (resulting string=w566:string)  [unwired: 2 in, 1 out]
                      }
                      frame False {
                        n110 = Format Into String(format string=w573, w575, w570, 1 ("BREAKDOWN_STK_HOLD_ID"), w572) -> (resulting string=w571:string)  [unwired: 2 in, 1 out]
                      }
                    }
                    n111 = call "Execute query.vi"("error in (no error)"=w564, "String"=w549, "connection reference"=w563) -> ("error out"=w556:errorcluster, "Table"=w562:string[][], "connection reference 2"=w559:T2)  [unwired: 5 in, 1 out]
                    n112 = call "monthwise_bd_summery.vi"("O/P 3"=w554, "error in (no error)"=w556, "Table"=w562) -> ("error out"=w555:errorcluster, "O/P 2"=w558:string[], "O/P"=w557:string[])  [unwired: 6 in]
                  }
                  frame #1 {
                    n113 = case shown="True" w577 {
                      tunnel: [w597 w603] -> w590
                      tunnel: w582 -> [w596 w602]
                      tunnel: w580 -> [_ _]
                      tunnel: w579 -> [w595 w601]
                      tunnel: w578 -> [_ w600]
                      tunnel: w576 -> [w594 w599]
                      frame True {
                        n114 = Format Into String(format string=w595, w596, w594, 2 ("BREAKDOWN_STK_HOLD_ID")) -> (resulting string=w597:string)  [unwired: 2 in, 1 out]
                      }
                      frame False {
                        n115 = Format Into String(format string=w601, w602, w599, 2 ("BREAKDOWN_STK_HOLD_ID"), w600) -> (resulting string=w603:string)  [unwired: 2 in, 1 out]
                      }
                    }
                    n116 = call "Execute query.vi"("error in (no error)"=w591, "String"=w590, "connection reference"=w592) -> ("error out"=w593:errorcluster, "Table"=w589:string[][], "connection reference 2"=w584:T2)  [unwired: 5 in, 1 out]
                    n117 = call "monthwise_bd_summery.vi"("O/P 3"=w581, "error in (no error)"=w593, "Table"=w589) -> ("error out"=w583:errorcluster, "O/P 2"=w586:string[], "O/P"=w585:string[])  [unwired: 6 in]
                  }
                  frame #2 {
                    n118 = case shown="True" w608 {
                      tunnel: [w628 w634] -> w609
                      tunnel: w611 -> [w627 w633]
                      tunnel: w607 -> [_ _]
                      tunnel: w610 -> [_ w632]
                      tunnel: w606 -> [w626 w631]
                      tunnel: w605 -> [w625 w630]
                      frame True {
                        n119 = Format Into String(format string=w626, w627, w625, 3 ("BREAKDOWN_STK_HOLD_ID")) -> (resulting string=w628:string)  [unwired: 2 in, 1 out]
                      }
                      frame False {
                        n120 = Format Into String(format string=w631, w633, w630, 3 ("BREAKDOWN_STK_HOLD_ID"), w632) -> (resulting string=w634:string)  [unwired: 2 in, 1 out]
                      }
                    }
                    n121 = call "Execute query.vi"("error in (no error)"=w617, "String"=w609, "connection reference"=w618) -> ("error out"=w619:errorcluster, "Table"=w620:string[][], "connection reference 2"=w613:T2)  [unwired: 5 in, 1 out]
                    n122 = call "monthwise_bd_summery.vi"("O/P 3"=w612, "error in (no error)"=w619, "Table"=w620) -> ("error out"=w614:errorcluster, "O/P 2"=w616:string[], "O/P"=w615:string[])  [unwired: 6 in]
                  }
                  frame #3 {
                    n123 = case shown="True" w637 {
                      tunnel: [w661 w667] -> w640
                      tunnel: w642 -> [_ w666]
                      tunnel: w638 -> [_ _]
                      tunnel: w641 -> [w659 w665]
                      tunnel: w639 -> [w660 w664]
                      tunnel: w636 -> [w658 w663]
                      frame True {
                        n124 = Format Into String(format string=w660, w659, w658, 4 ("BREAKDOWN_STK_HOLD_ID")) -> (resulting string=w661:string)  [unwired: 2 in, 1 out]
                      }
                      frame False {
                        n125 = Format Into String(format string=w664, w665, w663, 4 ("BREAKDOWN_STK_HOLD_ID"), w666) -> (resulting string=w667:string)  [unwired: 2 in, 1 out]
                      }
                    }
                    n126 = call "Execute query.vi"("error in (no error)"=w649, "String"=w640, "connection reference"=w648) -> ("error out"=w651:errorcluster, "Table"=w650:string[][], "connection reference 2"=w644:T2)  [unwired: 5 in, 1 out]
                    n127 = call "monthwise_bd_summery.vi"("O/P 3"=w643, "error in (no error)"=w651, "Table"=w650) -> ("error out"=w645:errorcluster, "O/P 2"=w647:string[], "O/P"=w646:string[])  [unwired: 6 in]
                  }
                  frame #4 {
                    n128 = case shown="True" w670 {
                      tunnel: [w696 w702] -> w675
                      tunnel: w674 -> [_ w701]
                      tunnel: w673 -> [w695 w700]
                      tunnel: w672 -> [w694 w699]
                      tunnel: w671 -> [_ _]
                      tunnel: w669 -> [w693 w698]
                      frame True {
                        n129 = Format Into String(format string=w695, w694, w693, 5 ("BREAKDOWN_STK_HOLD_ID")) -> (resulting string=w696:string)  [unwired: 2 in, 1 out]
                      }
                      frame False {
                        n130 = Format Into String(format string=w700, w699, w698, 5 ("BREAKDOWN_STK_HOLD_ID"), w701) -> (resulting string=w702:string)  [unwired: 2 in, 1 out]
                      }
                    }
                    n131 = call "Execute query.vi"("error in (no error)"=w682, "String"=w675, "connection reference"=w681) -> ("error out"=w683:errorcluster, "Table"=w684:string[][], "connection reference 2"=w678:T2)  [unwired: 5 in, 1 out]
                    n132 = call "monthwise_bd_summery.vi"("O/P 3"=w676, "error in (no error)"=w683, "Table"=w684) -> ("error out"=w677:errorcluster, "O/P 2"=w680:string[], "O/P"=w679:string[])  [unwired: 6 in]
                  }
                  frame #5 {
                    n133 = call "String to numeric.vi"("Array"=w738) -> ("Array 2"=w708:dbl[])  [unwired: 4 in]
                    n134 = call "String to numeric.vi"("Array"=w737) -> ("Array 2"=w707:dbl[])  [unwired: 4 in]
                    n135 = call "String to numeric.vi"("Array"=w736) -> ("Array 2"=w706:dbl[])  [unwired: 4 in]
                    n136 = call "String to numeric.vi"("Array"=w735) -> ("Array 2"=w704:dbl[])  [unwired: 4 in]
                    n137 = call "String to numeric.vi"("Array"=w734) -> ("Array 2"=w705:dbl[])  [unwired: 4 in]
                    n138 = Decimal String To Number(string=w713) -> (number=w718:i32[])  [unwired: 2 in, 1 out]
                    n139 = Decimal String To Number(string=w712) -> (number=w717:i32[])  [unwired: 2 in, 1 out]
                    n140 = Decimal String To Number(string=w711) -> (number=w716:i32[])  [unwired: 2 in, 1 out]
                    n141 = Decimal String To Number(string=w710) -> (number=w715:i32[])  [unwired: 2 in, 1 out]
                    n142 = Decimal String To Number(string=w709) -> (number=w714:i32[])  [unwired: 2 in, 1 out]
                    n143 = Compound Arithmetic op=ADD(w708, w707, w706, w704, w705) -> (w720:dbl[])
                    n144 = for {
                      tunnel: w720 -> [w746] mode=indexing
                      tunnel: [w745] -> w719 mode=indexing
                      n145 = Format Value(format string="%<%H:%M:%S>t", value (0)=w746) -> (output string=w745:string)  [unwired: 1 in]
                    }
                    n146 = Build Array(w738) -> (w744:string[][])
                    n147 = Build Array(w737) -> (w743:string[][])
                    n148 = Build Array(w736) -> (w742:string[][])
                    n149 = Build Array(w735) -> (w741:string[][])
                    n150 = Build Array(w734) -> (w740:string[][])
                    n151 = Build Array(w723) -> (w732:string[][])
                    n152 = Transpose 2D Array(2D array=w744) -> (transposed array=w730:string[][])
                    n153 = Transpose 2D Array(2D array=w743) -> (transposed array=w729:string[][])
                    n154 = Transpose 2D Array(2D array=w742) -> (transposed array=w728:string[][])
                    n155 = Transpose 2D Array(2D array=w741) -> (transposed array=w727:string[][])
                    n156 = Transpose 2D Array(2D array=w740) -> (transposed array=w726:string[][])
                    n157 = Transpose 2D Array(2D array=w732) -> (transposed array=w731:string[][])
                    n158 = Build Array(w719) -> (w739:string[][])
                    n159 = Compound Arithmetic op=ADD(w718, w717, w716, w715, w714) -> (w733:i32[])
                    n160 = Transpose 2D Array(2D array=w739) -> (transposed array=w724:string[][])
                    n161 = Number To Decimal String(number=w733) -> (decimal integer string=w725:string[])  [unwired: 1 in]
                  }
                  frame #6 {
                    n162 = Add Array Elements(numeric array=w752) -> (sum=w765:dbl)
                    n163 = Add Array Elements(numeric array=w751) -> (sum=w766:dbl)
                    n164 = Add Array Elements(numeric array=w750) -> (sum=w767:dbl)
                    n165 = Add Array Elements(numeric array=w748) -> (sum=w768:dbl)
                    n166 = Add Array Elements(numeric array=w749) -> (sum=w769:dbl)
                    n167 = Add Array Elements(numeric array=w757) -> (sum=w763:i32)
                    n168 = Add Array Elements(numeric array=w756) -> (sum=w762:i32)
                    n169 = Add Array Elements(numeric array=w755) -> (sum=w761:i32)
                    n170 = Add Array Elements(numeric array=w754) -> (sum=w760:i32)
                    n171 = Add Array Elements(numeric array=w753) -> (sum=w759:i32)
                    n172 = Insert Into Array(array=w824, index (col)=1 ("disabled index (col)"), new element #1=w823, new element #2=w822, new element #3=w821, new element #4=w820, new element #5=w819, new element #6=w818, new element #7=w817, new element #8=w816, new element #9=w815, new element #10=w814, new element #11=w812, new element #12=w813) -> (w811:string[][])  [unwired: 1 in]
                    "Table Control" <- w811
                    n173 = Build Array(w765, w766, w767, w768, w769) -> (w764:dbl[])
                    n174 = Build Array(w763, w762, w761, w760, w759) -> (w758:i32[])
                    n175 = call-poly <vilib>:"Plot Helper.vi"("x vector"=w758) -> ("error out"=w773:errorcluster, "3D Plot lvclass Array out"=→"Count 2":refnum<class "3D Plot Datatype.lvclass">[])  [unwired: 2 in, 7 out]
                    n176 = call-poly <vilib>:"Plot Helper.vi"("x vector"=w764) -> ("error out"=w771:errorcluster, "3D Plot lvclass Array out"=→"Duration":refnum<class "3D Plot Datatype.lvclass">[])  [unwired: 2 in, 7 out]
                    n177 = Index Array(array=w811, index (col) #1=1 ("disabled index (col)")) -> (element #1=w809:string[], element #2=w808:string[], element #3=w807:string[], element #4=w806:string[], element #5=w805:string[], element #6=w804:string[], element #7=w803:string[], element #8=w802:string[], element #9=w801:string[], element #10=w800:string[], element #11=w799:string[], element #12=w798:string[])  [unwired: 23 in]
                    n178 = disable-structure shown="Enabled" {
                      disable-tunnel: w809 -> [w849 w861]
                      disable-tunnel: w808 -> [w848 w873]
                      disable-tunnel: w807 -> [w847 w854]
                      disable-tunnel: w806 -> [w846 w871]
                      disable-tunnel: w805 -> [w845 w855]
                      disable-tunnel: w804 -> [w844 w869]
                      disable-tunnel: w803 -> [w843 w856]
                      disable-tunnel: w802 -> [w842 w867]
                      disable-tunnel: w801 -> [w841 w857]
                      disable-tunnel: w800 -> [w840 w866]
                      disable-tunnel: w799 -> [w839 w858]
                      disable-tunnel: w798 -> [w838 w865]
                      disable-tunnel: [w837 w860] -> w797
                      disable-tunnel: [w836 w853] -> w796
                      disable-tunnel: [w835 w852] -> w795
                      disable-tunnel: [w834 w859] -> w794
                      disable-tunnel: [w833 w851] -> w793
                      disable-tunnel: [w832 w850] -> w792
                      disable-tunnel: [w831 w872] -> w791
                      disable-tunnel: [w830 w870] -> w790
                      disable-tunnel: [w829 w868] -> w789
                      disable-tunnel: [w828 w862] -> w788
                      disable-tunnel: [w827 w863] -> w787
                      disable-tunnel: [w826 w864] -> w786
                      frame Disabled {
                        n179 = call "SUM_ARRAY.vi"("Array"=w849) -> ("F-format string"=w837:string)  [unwired: 6 in]
                        n180 = call "SUM_ARRAY.vi"("Array"=w848) -> ("F-format string"=w831:string)  [unwired: 6 in]
                        n181 = call "SUM_ARRAY.vi"("Array"=w847) -> ("F-format string"=w836:string)  [unwired: 6 in]
                        n182 = call "SUM_ARRAY.vi"("Array"=w846) -> ("F-format string"=w830:string)  [unwired: 6 in]
                        n183 = call "SUM_ARRAY.vi"("Array"=w845) -> ("F-format string"=w835:string)  [unwired: 6 in]
                        n184 = call "SUM_ARRAY.vi"("Array"=w844) -> ("F-format string"=w829:string)  [unwired: 6 in]
                        n185 = call "SUM_ARRAY.vi"("Array"=w843) -> ("F-format string"=w834:string)  [unwired: 6 in]
                        n186 = call "SUM_ARRAY.vi"("Array"=w842) -> ("F-format string"=w828:string)  [unwired: 6 in]
                        n187 = call "SUM_ARRAY.vi"("Array"=w841) -> ("F-format string"=w833:string)  [unwired: 6 in]
                        n188 = call "SUM_ARRAY.vi"("Array"=w840) -> ("F-format string"=w827:string)  [unwired: 6 in]
                        n189 = call "SUM_ARRAY.vi"("Array"=w839) -> ("F-format string"=w832:string)  [unwired: 6 in]
                        n190 = call "SUM_ARRAY.vi"("Array"=w838) -> ("F-format string"=w826:string)  [unwired: 6 in]
                      }
                      frame Enabled {
                        n191 = call "SUM_ARRAY.vi"("Array"=w861) -> ("F-format string"=w860:string)  [unwired: 6 in]
                        n192 = call "time string to minutes string.vi"("Array"=w873) -> ("output string"=w872:string)  [unwired: 10 in]
                        n193 = call "SUM_ARRAY.vi"("Array"=w854) -> ("F-format string"=w853:string)  [unwired: 6 in]
                        n194 = call "time string to minutes string.vi"("Array"=w871) -> ("output string"=w870:string)  [unwired: 10 in]
                        n195 = call "SUM_ARRAY.vi"("Array"=w855) -> ("F-format string"=w852:string)  [unwired: 6 in]
                        n196 = call "time string to minutes string.vi"("Array"=w869) -> ("output string"=w868:string)  [unwired: 10 in]
                        n197 = call "SUM_ARRAY.vi"("Array"=w856) -> ("F-format string"=w859:string)  [unwired: 6 in]
                        n198 = call "time string to minutes string.vi"("Array"=w867) -> ("output string"=w862:string)  [unwired: 10 in]
                        n199 = call "SUM_ARRAY.vi"("Array"=w857) -> ("F-format string"=w851:string)  [unwired: 6 in]
                        n200 = call "time string to minutes string.vi"("Array"=w866) -> ("output string"=w863:string)  [unwired: 10 in]
                        n201 = call "SUM_ARRAY.vi"("Array"=w858) -> ("F-format string"=w850:string)  [unwired: 6 in]
                        n202 = call "time string to minutes string.vi"("Array"=w865) -> ("output string"=w864:string)  [unwired: 10 in]
                      }
                    }
                    n203 = Unbundle By Name(w773) -> ()  [unwired: 1 out]
                    n204 = Unbundle By Name(w771) -> ()  [unwired: 1 out]
                    n205 = call "Plot PieChart.vi"("Label"=string[] ["Safety", "Material", "Maintenance", "Quality", "Startup_Setup"]) -> ("Labelling"=w776:cluster{dbl, "String":string}[])  [unwired: 10 in]
                    n206 = call "CONCATINATE_STRING.vi"("F-format string"=w790, "F-format string 2"=w796) -> ("concatenated string"=→"L":string)  [unwired: 9 in]
                    n207 = call "CONCATINATE_STRING.vi"("F-format string"=w789, "F-format string 2"=w795) -> ("concatenated string"=→"M":string)  [unwired: 9 in]
                    n208 = call "CONCATINATE_STRING.vi"("F-format string"=w788, "F-format string 2"=w794) -> ("concatenated string"=→"Q":string)  [unwired: 9 in]
                    n209 = call "CONCATINATE_STRING.vi"("F-format string"=w787, "F-format string 2"=w793) -> ("concatenated string"=→"P":string)  [unwired: 9 in]
                    n210 = call "CONCATINATE_STRING.vi"("F-format string"=w791, "F-format string 2"=w797) -> ("concatenated string"=→"GL":string)  [unwired: 9 in]
                    n211 = call "CONCATINATE_STRING.vi"("F-format string"=w786, "F-format string 2"=w792) -> ("concatenated string"=→"T":string)  [unwired: 9 in]
                    n212 = property on="Duration" class="3D Pie (strict)"("Plot Specific:Color and Name"=w776) -> (error out=w775:errorcluster)  [unwired: 2 in, 1 out]
                    n213 = property on="Count 2" class="3D Pie (strict)"("Plot Specific:Color and Name"=w776) -> (error out=w774:errorcluster)  [unwired: 2 in, 1 out]
                    n214 = Unbundle By Name(w775) -> ()  [unwired: 1 out]
                    n215 = Unbundle By Name(w774) -> ()  [unwired: 1 out]
                    "O/P 4" <- w823
                  }
                }
              }
            }
          }
        }
      }
      event "Download 2": Value Change {
        n216 = event-data() -> ()  [unwired: 1 in, 6 out]
        n217 = local read "Table Control"() -> (w887:string[][])
        n218 = Empty Array?(array=w887) -> (empty?=w888:bool)
        n219 = case shown="False" w888 {
          tunnel: w887 -> [w906 _]
          tunnel: w890 -> [w905 w915]
          tunnel: [w904 w915] -> w889
          frame False {
            w900 = 1 ("index (row)")
            n220 = local read "Select Station"() -> (w895:string)
            n221 = local read "Select Month"() -> (w897:string)
            n222 = case shown="\"ALL\", Default" w895 {
              tunnel: ["All" "250T-3" "250T-2" "250T-1" "400T-1" "150T-1" "400T-2"] -> w898
              frame "ALL", Default {
              }
              frame "ST 1" {
              }
              frame "ST 2" {
              }
              frame "ST 3" {
              }
              frame "ST 4" {
              }
              frame "ST 5" {
              }
              frame "ST 6" {
              }
            }
            n223 = local read "Select Year"() -> (w896:string)
            n224 = local read "Shift"() -> (w894:string)
            n225 = Replace Array Subset(array=string[][] [["L&L Products", "Breakdown Summary", "Monthwise", "", "", "", "", "", "", "", "", "", ""], ["Month:", "", "Year:", "", "Station:", "", "Shift:", "", "", "", "", "", ""], ["", "", "", "", "", "", "", "", "", "", "", "", ""], ["Date", "Safety Count", "Duration", "Material Count", "Duration", "Maintenance Count", "Duration", "Quality Count", "Duration", "Startup_Setup Count", "Duration", "Total Count", "Duration"]] ("Column Header Strings[]"), new element #1=w897, index (row) #1=w900, index (col) #1=w900, new element #2=w896, index (row) #2=w900, index (col) #2=3 ("disabled index (col)"), new element #3=w898, index (row) #3=w900, index (col) #3=5 ("disabled index (col)"), new element #4=w894, index (row) #4=w900, index (col) #4=7 ("disabled index (col)")) -> (w893:string[][])
            n226 = call "Download_Report_subvi.vi"("error in (no error)"=w905, "Value"=w906, "Column Header Strings[]"=w893) -> ("error out"=w904:errorcluster)  [unwired: 8 in]
          }
          frame True {
            n227 = One Button Dialog(message="No record found!") -> ()  [unwired: 1 in, 1 out]
          }
        }
      }
      event "Cancel Button - Archive": Value Change {
        n228 = event-data() -> ()  [unwired: 1 in, 6 out]
      }
    }
    n229 = Wait (ms)(milliseconds to wait=u32 50) -> ()  [unwired: 1 out]
  }
  n230 = call <vilib>:"DB Tools Close Connection.vi"("error in (no error)"=w4, "connection reference"=w5) -> ("error out"=w3:errorcluster)  [unwired: 5 in]
  n231 = call <vilib>:"Clear Errors.vi"("error in (no error)"=w3) -> ("error out"=w9:errorcluster)  [unwired: 5 in, 1 out]
  n232 = property class="App"(error in=w9) -> (error out=w8:errorcluster, "App.Kind"=w7:T3)  [unwired: 1 in, 1 out]
  n233 = case shown="\"Development System\", Default" w7 {
    tunnel: w8 -> [w920 w922]
    tunnel: [w919 w921] -> w6
    frame "Development System", Default {
      n234 = invoke class="VI" method="FP.Close"(error in=w920) -> (error out=w919:errorcluster)  [unwired: 2 in, 2 out]
    }
    frame "Run Time System" {
      n235 = invoke class="VI" method="FP.Close"(error in=w922) -> (error out=w921:errorcluster)  [unwired: 2 in, 2 out]
    }
  }
  "error out" <- w6
